vi "Autonics_1Scan.vi"() -> ()   [LabVIEW 2018]
uses:
  <vilib>/Platform/NI_3dgraph.lvlib
  <vilib>/Utility/file.llb/Write To Spreadsheet File (DBL).vi
  <vilib>/DAQmx/read.llb/DAQmx Read (Analog 2D DBL NChan NSamp).vi
  <resource>/objmgr/daqmx.rc
  <vilib>/Instr/_visa.llb/VISA Configure Serial Port (Instr).vi
  <vilib>/Utility/file.llb/Read From Spreadsheet File (DBL).vi
  <vilib>/DAQmx/configure/timing.llb/DAQmx Timing (Sample Clock).vi
  <vilib>/DAQmx/create/channels.llb/DAQmx Create Channel (AI-Voltage-Basic).vi
  <vilib>/Analysis/Matrix/Datatypes/RealMatrix.ctl
  <vilib>/Analysis/Matrix/NI_Matrix.lvlib
panel:
  out "Numeric 2":i32
  out "Numeric":i32
  out "Process Output (Matrix)":T1
  out "Waveform Graph":dbl[](graph)
  in  "Selected Scanning Channel":dbl
  in  "Display Scanning Channel":bool
  out "Waveform Chart":dbl[][](graph)
  in  "Test Channel":bool
  in  "Open":bool
  in  "Scan Distance":dbl=457.0
  in  "Multiplier":dbl=10.0
  in  "Save Button":bool
  in  "No Save":bool
  in  "Save Link":path
  in  "ViewMode":i32(ring) items=["cwViewXYPlane", "cwViewXZPlane", "cwViewYZPlane", "cwViewUserDefined"]
  in  "Back data":bool
  in  "Data Type":u16(ring)=1 items=["Normal", "dX", "dY"]
  in  "Sampling Rate(Hz)":dbl=15000.0
  in  "Samples per Channels":i32=1000
  in  "Min Volts":dbl=-10.0 format="%0.2f"
  in  "Max Volts":dbl=10.0 format="%0.2f"
  in  "Channels":tag="Dev2/ai0:67"
  in  "Scan Step (mm)":dbl=1.0
  in  "Scan":bool
  in  "Plot style":i32(ring)=5 items=["cwLine"=1, "cwPoint"=2, "cwLinePoint"=3, "cwHiddenLine"=4, "cwSurface"=5, "cwSurfaceLine"=6, "cwSurfaceNormal"=7, "cwContourLine"=8, "cwSurfaceContour"=9]
  in  "3D Surface":refnum<k7>(container)
  in  "Flow control":u16(ring) items=["None", "XON/XOFF", "RTS/CTS", "XON/XOFF & RTS/CTS", "DTR/DSR", "XON/XOFF & DTR/DSR"]
  in  "Stop bits":u16(ring)=10 items=["1.0"=10, "1.5"=15, "2.0"=20]
  in  "Parity":dbl
  in  "Data bits":u16=8 min=5 max=8 step=1
  in  "Baud Rate":u32=57600
  in  "COM Port":refnum<visa-resource-name>="COM3"
  in  "Travel per Pulse (mm)":dbl=0.002
  in  "Speed (mm/s)":dbl=5.0
  out "Current  Position (mm)":dbl format="%#_4g"
  in  "Move Distance (mm)":dbl=1.0
  in  "Stop Scan":bool
  in  "Stop":bool
  in  "Home":bool
  in  "Right":bool
  in  "Left":bool
  # "SCANER CONTROL"
  # "BOBBIN MAGNETIC CAMERA"
  # "CHANNELS"
  # "COM Setting"
  # "TIMING"
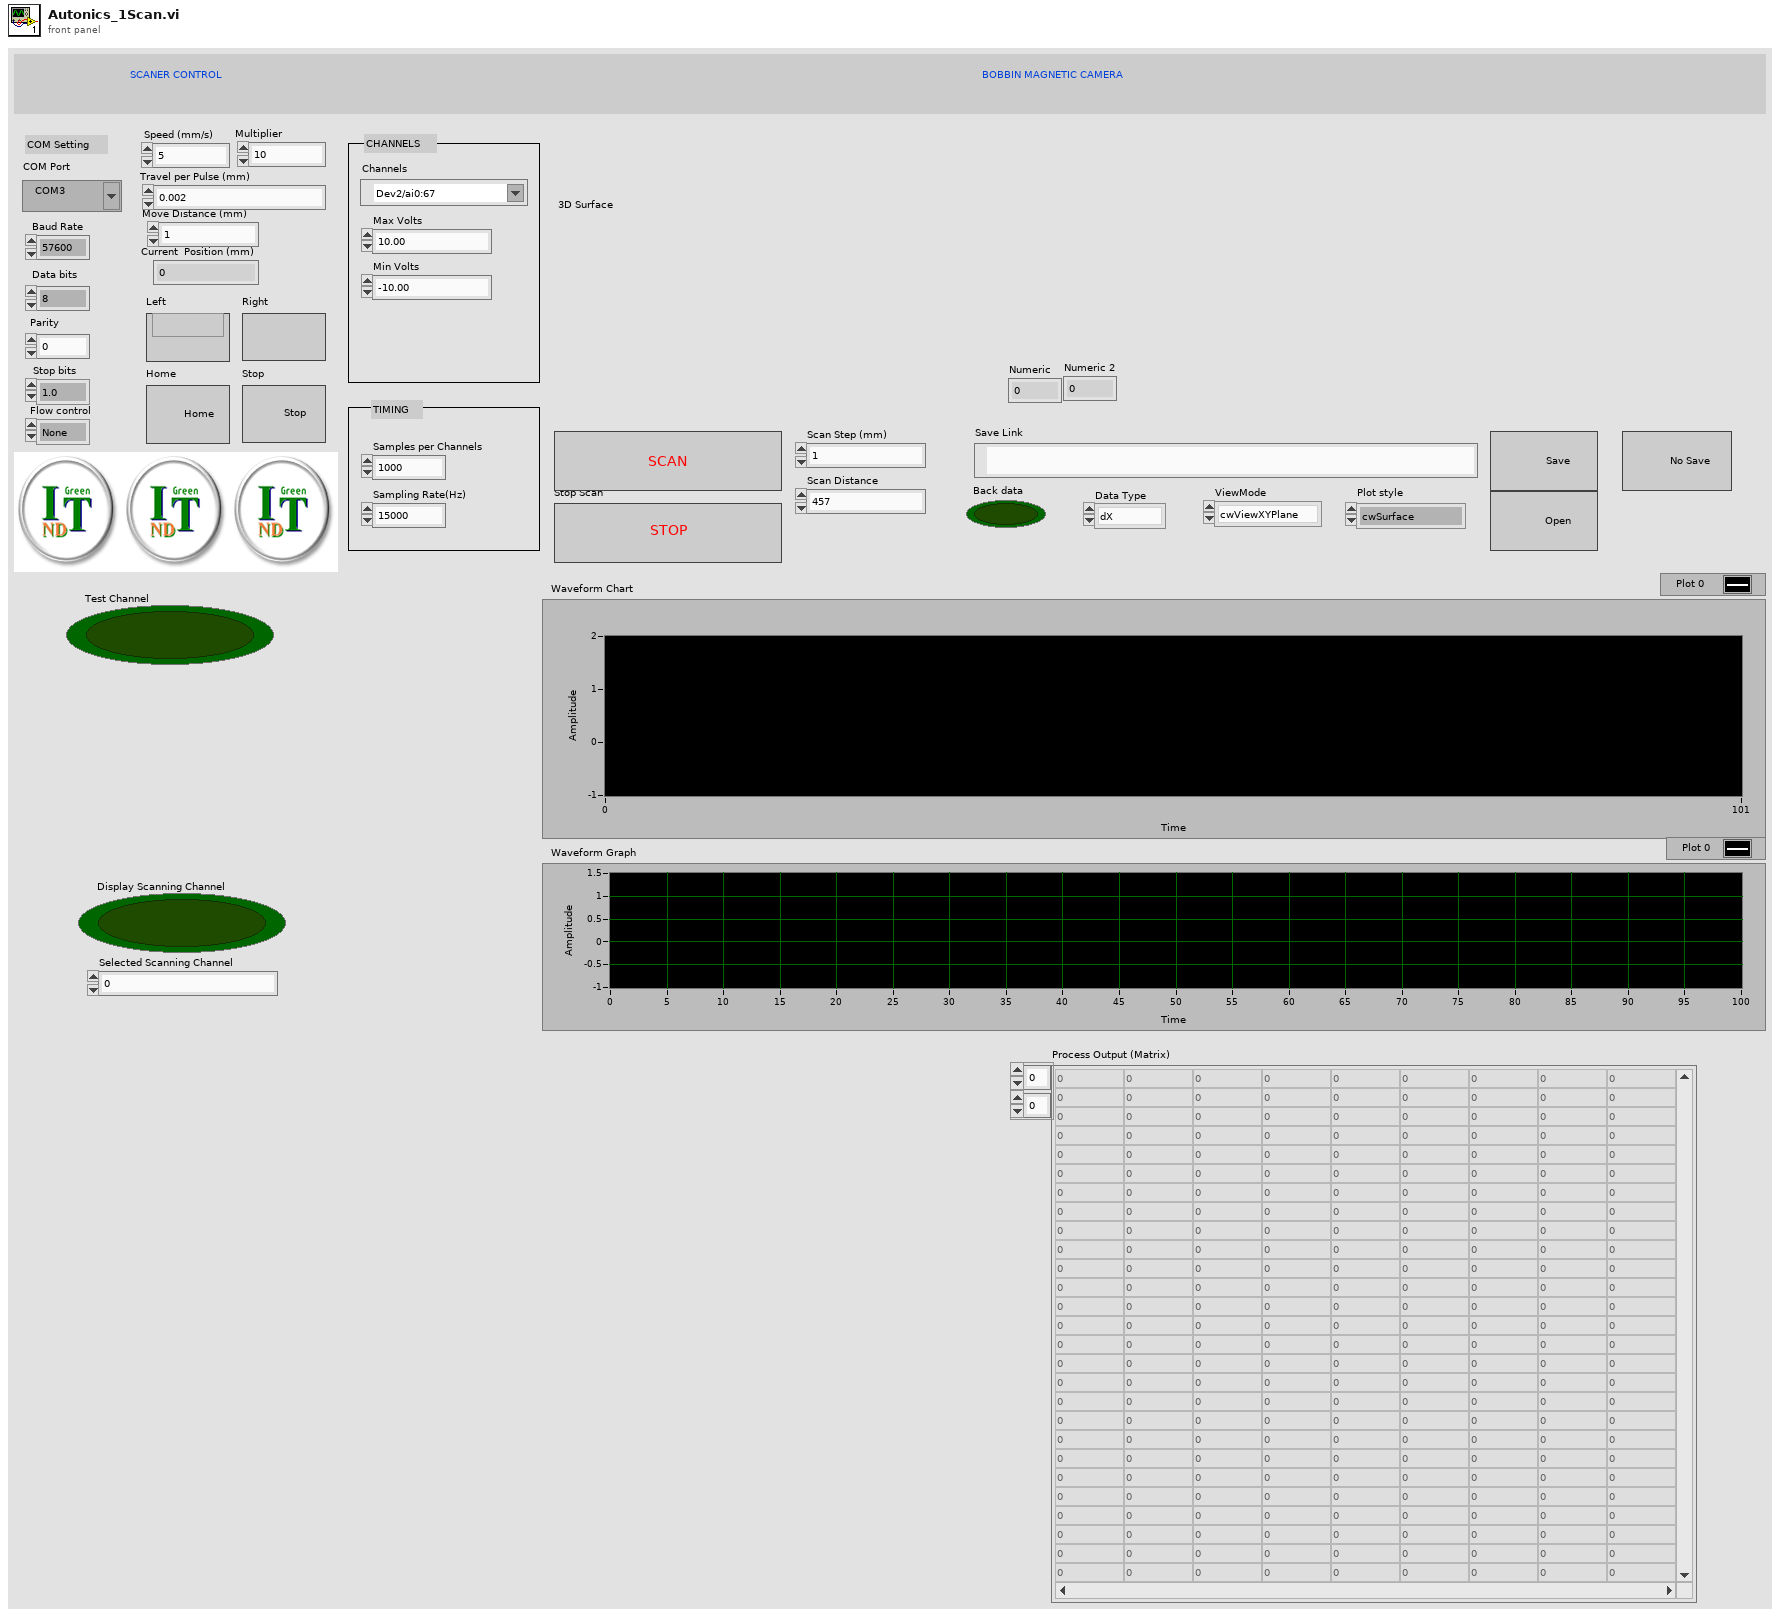
[diagram p1: front panel]
types:
  T1 = typedef "NI_Matrix.lvlib/RealMatrix.ctl" = dbl[][]
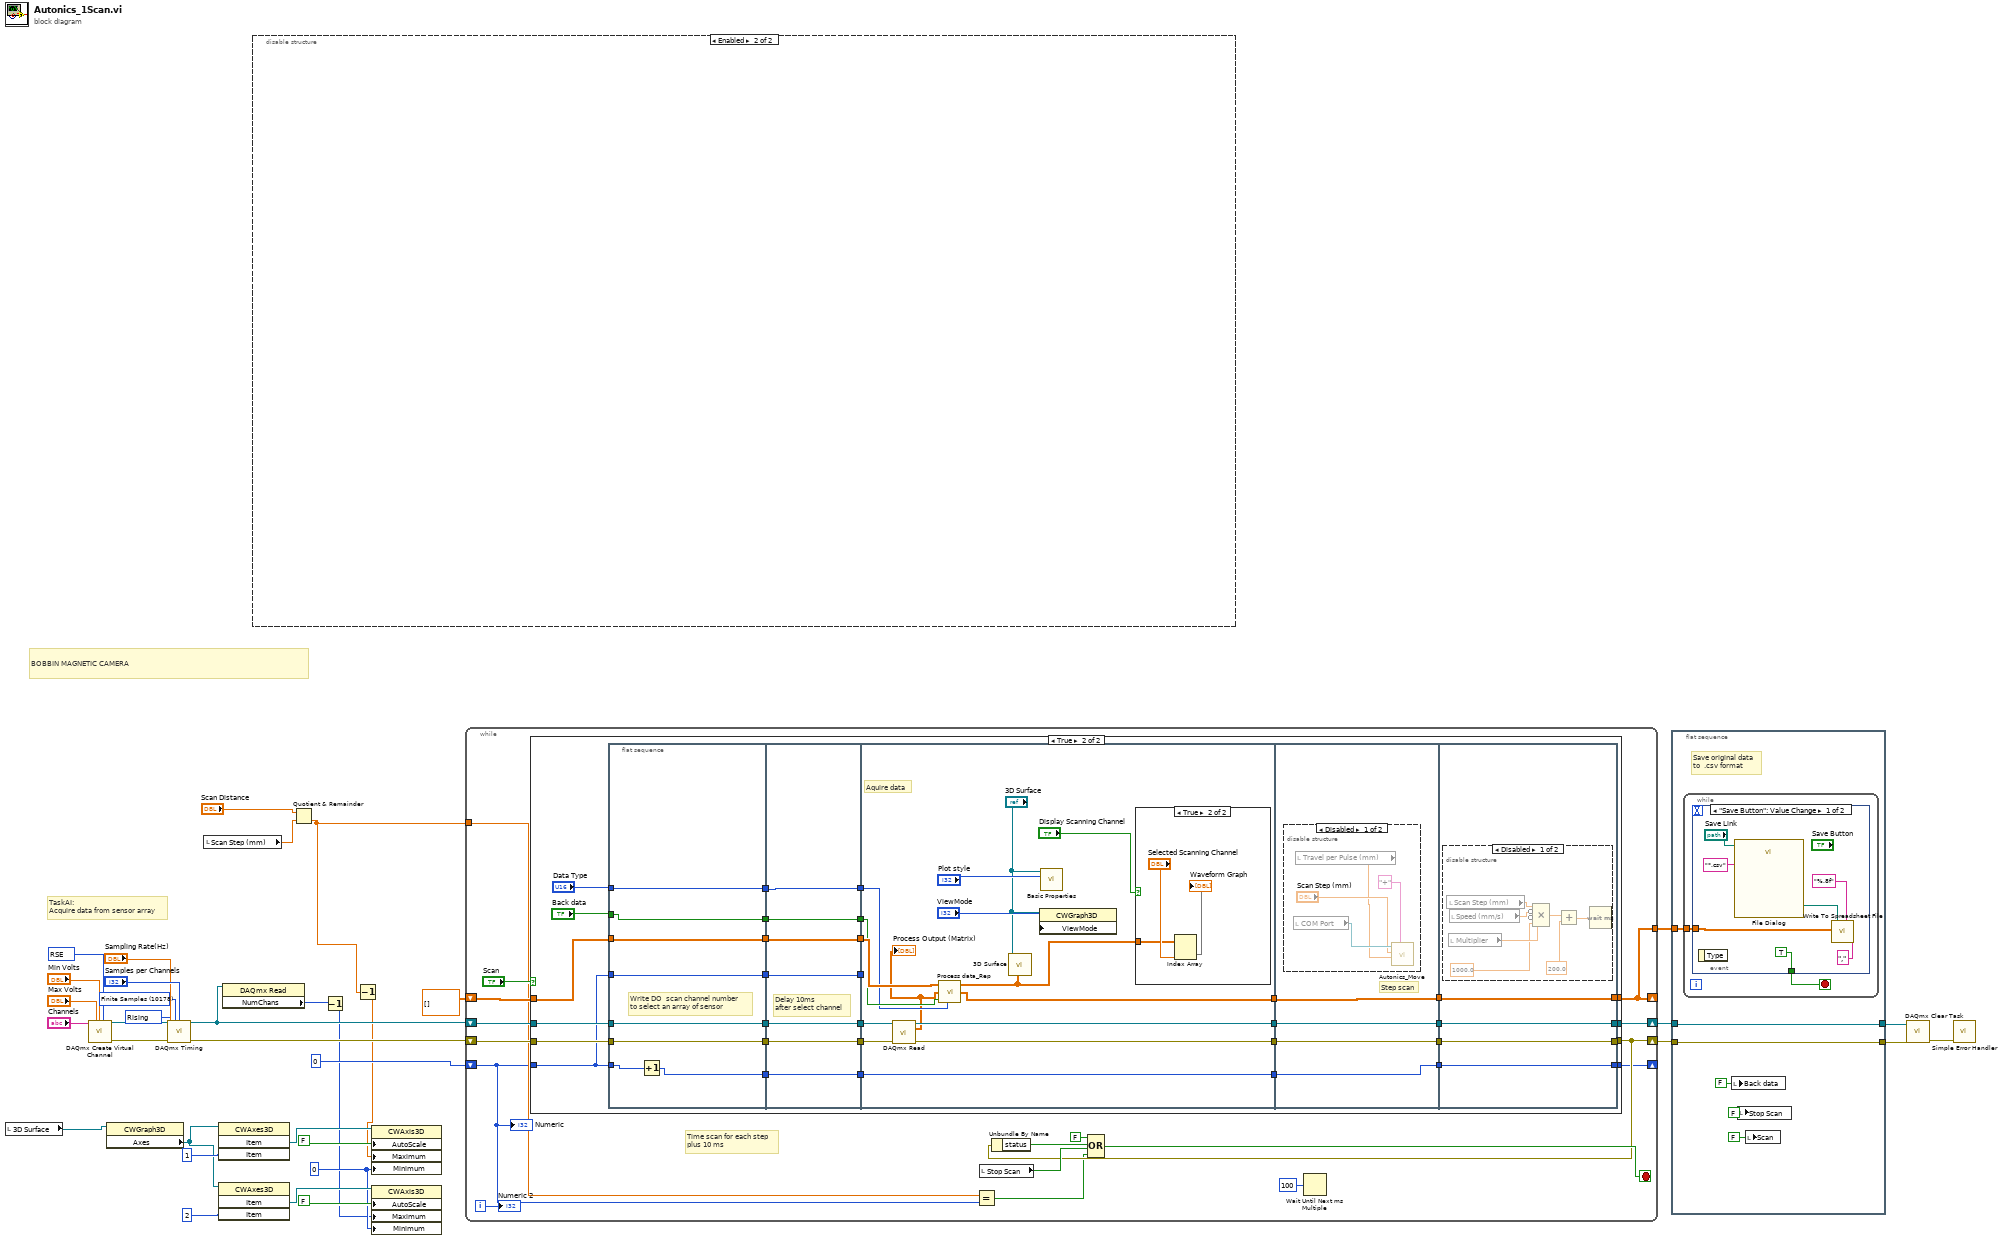
[diagram p0: block diagram]
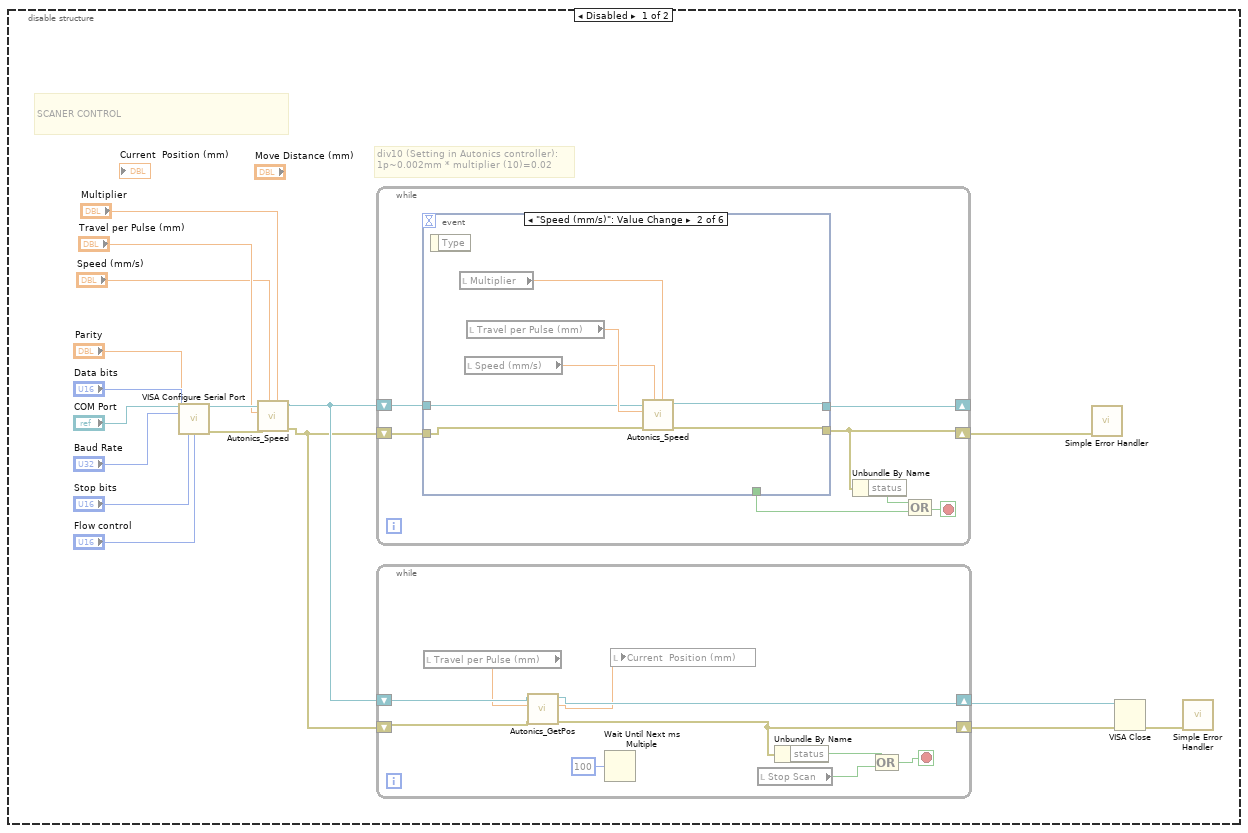
[diagram p2: hidden frame]
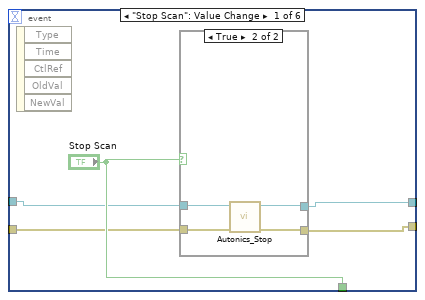
[diagram p3: hidden frame]
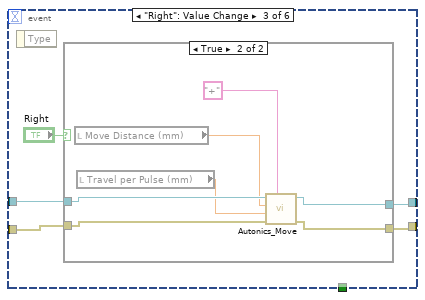
[diagram p5: hidden frame]
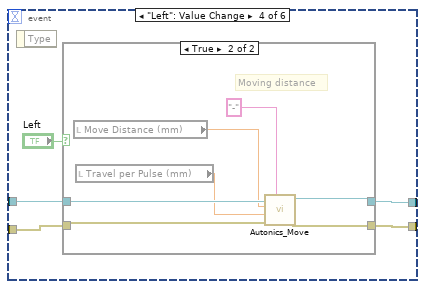
[diagram p7: hidden frame]
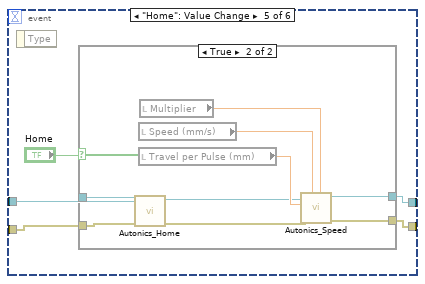
[diagram p9: hidden frame]
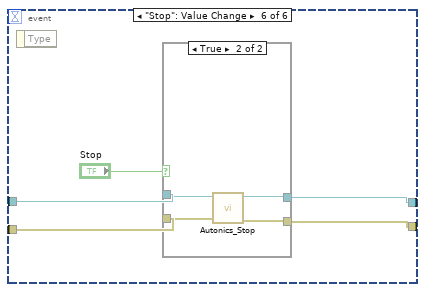
[diagram p11: hidden frame]
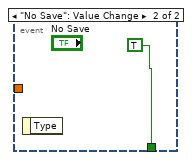
[diagram p13: hidden frame]
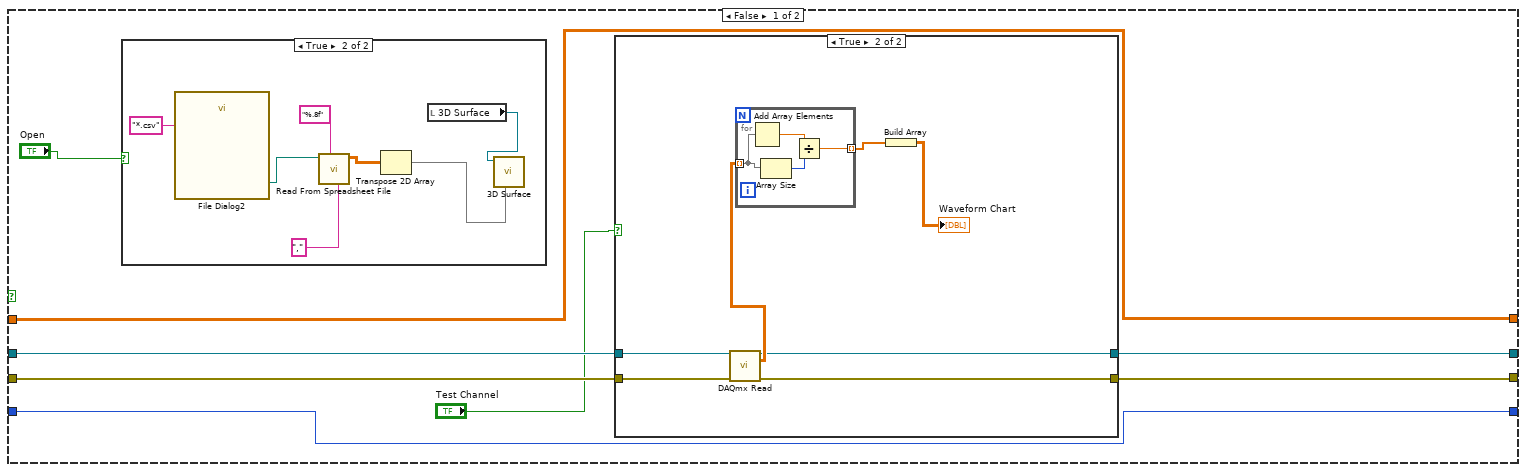
[diagram p14: hidden frame]
diagram:
  w2 = 10280 items=["Rising"=10280, "Falling"=10171] ("active edge")
  w13 = 0
  w26 = 10083 items=["default"=-1, "RSE"=10083, "NRSE"=10078, "Differential"=10106, "Pseudodifferential"=12529] ("input terminal configuration")
  w27 = 10178 items=["Finite Samples"=10178, "Continuous Samples"=10123, "Hardware Timed Single Point"=12522] ("sample mode")
  # "TaskAI:\nAcquire data from sensor array"
  # "BOBBIN MAGNETIC CAMERA"
  n1 = local read "3D Surface"() -> (w21:refnum<k7>)
  n2 = call-poly <vilib>:"DAQmx Create Virtual Channel.vi"("maximum value"="Max Volts", "minimum value"="Min Volts", "input terminal configuration"=w26, "physical channels"="Channels") -> ("task out"=w35:refnum<k21>, "error out"=w34:errorcluster)  [unwired: 10 in]
  n3 = property class="CWGraph3D"(reference=w21) -> ("Axes"=w14:refnum<k7>)  [unwired: 1 in, 2 out]
  n4 = call-poly <vilib>:"DAQmx Timing.vi"("task/channels in"=w35, "sample mode"=w27, "samples per channel"="Samples per Channels", "rate"="Sampling Rate(Hz)", "active edge"=w2, "error in"=w34) -> ("task out"=w25:refnum<k21>, "error out"=w28:errorcluster)  [unwired: 8 in]
  n5 = local read "Scan Step (mm)"() -> (w24:dbl)
  n6 = invoke class="CWAxes3D" method="Item"(reference=w14, "Item"=1) -> ("Item"=w20:refnum<k7>)  [unwired: 2 in, 3 out]
  n7 = invoke class="CWAxes3D" method="Item"(reference=w14, "Item"=2) -> ("Item"=w15:refnum<k7>)  [unwired: 2 in, 3 out]
  n8 = property class="DAQmx Read"(reference=w25) -> ("NumChans"=w4:u32)  [unwired: 1 in, 2 out]
  n9 = disable-structure shown="Enabled" {
    frame Disabled {
      # "div10 (Setting in Autonics controller):\n1p~0.002mm * multiplier (10)=0.02"
      # "SCANER CONTROL"
      n10 = call-poly "VISA Configure Serial Port"("VISA resource name"="COM Port", "baud rate (9600)"="Baud Rate", "data bits (8)"="Data bits", "parity (0:none)"="Parity", "stop bits (10: 1 bit)"="Stop bits", "flow control (0:none)"="Flow control") -> ("VISA resource name out"=w40:refnum<visa-resource-name>, "error out"=w39:errorcluster)  [unwired: 8 in]
      n11 = call "Autonics_Speed.vi"("Multiplier"="Multiplier", "Speed (mm/s)"="Speed (mm/s)", "error in (no error)"=w39, "Travel per  Pulse"="Travel per Pulse (mm)", "VISA resource name"=w40) -> ("error out"=w41:errorcluster, "VISA resource name out"=w42:refnum<visa-resource-name>)  [unwired: 5 in]
      n12 = while {
        shift-right: [w69] -> _
        shift-left: w42 -> [w68]
        shift-right: [w65] -> w45
        shift-left: w41 -> [w67]
        stop <- w64 stop-if-true
        n13 = event shown="[1] \"Speed (mm/s)\": Value Change" {
          selector: _ -> [_ _ _ _ _ _]
          dyn-events: _ -> [_ _ _ _ _ _]
          timeout: _ -> [_ _ _ _ _ _]
          tunnel: w68 -> [w73 w86 w90 w104 w120 w134]
          tunnel: w67 -> [w72 w85 w89 w103 w119 w133]
          tunnel: [w71 w84 w92 w106 w117 w136] -> w69
          tunnel: [w70 w83 w91 w105 w116 w135] -> w65
          tunnel: ["Stop Scan" _ _ _ _ _] -> w63
          event "Stop Scan": Value Change {
            n14 = event-data() -> ()  [unwired: 1 in, 5 out]
            n15 = case shown="True" "Stop Scan" {
              tunnel: [w76 w79] -> w71
              tunnel: [w75 w80] -> w70
              tunnel: w73 -> [w76 w78]
              tunnel: w72 -> [w75 w77]
              frame False {
              }
              frame True {
                n16 = call "Autonics_Stop.vi"("error in (no error)"=w77, "VISA resource name"=w78) -> ("error out"=w80:errorcluster, "VISA resource name out"=w79:refnum<visa-resource-name>)  [unwired: 8 in]
              }
            }
          }
          event "Speed (mm/s)": Value Change {
            n17 = event-data() -> ()  [unwired: 1 in, 1 out]
            n18 = local read "Multiplier"() -> (w81:dbl)
            n19 = local read "Speed (mm/s)"() -> (w82:dbl)
            n20 = local read "Travel per Pulse (mm)"() -> (w87:dbl)
            n21 = call "Autonics_Speed.vi"("Multiplier"=w81, "Speed (mm/s)"=w82, "error in (no error)"=w85, "Travel per  Pulse"=w87, "VISA resource name"=w86) -> ("error out"=w83:errorcluster, "VISA resource name out"=w84:refnum<visa-resource-name>)  [unwired: 5 in]
          }
          event "Right": Value Change {
            n22 = event-data() -> ()  [unwired: 1 in, 1 out]
            n23 = case shown="True" "Right" {
              tunnel: [w93 w99] -> w92
              tunnel: [w94 w98] -> w91
              tunnel: w90 -> [w93 w101]
              tunnel: w89 -> [w94 w100]
              frame False {
              }
              frame True {
                n24 = local read "Move Distance (mm)"() -> (w97:dbl)
                n25 = local read "Travel per Pulse (mm)"() -> (w96:dbl)
                n26 = call "Autonics_Move.vi"("Direction (+)"="+", "error in (no error)"=w100, "Travel per Pulse (mm)"=w96, "Move Distance (mm)"=w97, "VISA resource name"=w101) -> ("error out"=w98:errorcluster, "VISA resource name out"=w99:refnum<visa-resource-name>)  [unwired: 5 in]
              }
            }
          }
          event "Left": Value Change {
            n27 = event-data() -> ()  [unwired: 1 in, 1 out]
            n28 = case shown="True" "Left" {
              tunnel: [w108 w113] -> w106
              tunnel: [w107 w112] -> w105
              tunnel: w104 -> [w108 w115]
              tunnel: w103 -> [w107 w114]
              frame False {
              }
              frame True {
                # "Moving distance"
                n29 = local read "Move Distance (mm)"() -> (w110:dbl)
                n30 = local read "Travel per Pulse (mm)"() -> (w109:dbl)
                n31 = call "Autonics_Move.vi"("Direction (+)"="-", "error in (no error)"=w114, "Travel per Pulse (mm)"=w109, "Move Distance (mm)"=w110, "VISA resource name"=w115) -> ("error out"=w112:errorcluster, "VISA resource name out"=w113:refnum<visa-resource-name>)  [unwired: 5 in]
              }
            }
          }
          event "Home": Value Change {
            n32 = event-data() -> ()  [unwired: 1 in, 1 out]
            n33 = case shown="True" "Home" {
              tunnel: [w122 w124] -> w117
              tunnel: [w121 w123] -> w116
              tunnel: w120 -> [w122 w131]
              tunnel: w119 -> [w121 w130]
              frame False {
              }
              frame True {
                n34 = call "Autonics_Home.vi"("error in (no error)"=w130, "VISA resource name"=w131) -> ("error out"=w125:errorcluster, "VISA resource name out"=w126:refnum<visa-resource-name>)  [unwired: 8 in]
                n35 = local read "Speed (mm/s)"() -> (w128:dbl)
                n36 = local read "Travel per Pulse (mm)"() -> (w129:dbl)
                n37 = local read "Multiplier"() -> (w127:dbl)
                n38 = call "Autonics_Speed.vi"("Multiplier"=w127, "Speed (mm/s)"=w128, "error in (no error)"=w125, "Travel per  Pulse"=w129, "VISA resource name"=w126) -> ("error out"=w123:errorcluster, "VISA resource name out"=w124:refnum<visa-resource-name>)  [unwired: 5 in]
              }
            }
          }
          event "Stop": Value Change {
            n39 = event-data() -> ()  [unwired: 1 in, 1 out]
            n40 = case shown="True" "Stop" {
              tunnel: [w138 w139] -> w136
              tunnel: [w137 w142] -> w135
              tunnel: w134 -> [w138 w141]
              tunnel: w133 -> [w137 w140]
              frame False {
              }
              frame True {
                n41 = call "Autonics_Stop.vi"("error in (no error)"=w140, "VISA resource name"=w141) -> ("error out"=w142:errorcluster, "VISA resource name out"=w139:refnum<visa-resource-name>)  [unwired: 8 in]
              }
            }
          }
        }
        n42 = Unbundle By Name(w65) -> ("status"=w66:bool)
        n43 = Compound Arithmetic op=OR(w66, w63) -> (w64:bool)
      }
      n44 = while {
        shift-right: [w56] -> w44
        shift-left: w42 -> [w58]
        shift-right: [w55] -> w43
        shift-left: w41 -> [w57]
        stop <- w59 stop-if-true
        n45 = local read "Travel per Pulse (mm)"() -> (w54:dbl)
        n46 = call "Autonics_GetPos.vi"("error in (no error)"=w57, "Travel per Pulse (mm)"=w54, "VISA resource name"=w58) -> ("error out"=w55:errorcluster, "Current  Position (mm)"=w53:dbl, "VISA resource name out"=w56:refnum<visa-resource-name>)  [unwired: 6 in]
        n47 = Wait Until Next ms Multiple(millisecond multiple=u32 100) -> ()  [unwired: 1 out]
        n48 = local write "Current  Position (mm)"(w53) -> ()
        n49 = local read "Stop Scan"() -> (w60:bool)
        n50 = Unbundle By Name(w55) -> ("status"=w61:bool)
        n51 = Compound Arithmetic op=OR(w61, w60) -> (w59:bool)
      }
      n52 = call <vilib>:"Simple Error Handler.vi"("error in (no error)"=w45) -> ()  [unwired: 4 in, 5 out]
      n53 = VISA Close(VISA resource name=w44, error in (no error)=w43) -> (error out=w48:errorcluster)
      n54 = call <vilib>:"Simple Error Handler.vi"("error in (no error)"=w48) -> ()  [unwired: 4 in, 5 out]
    }
    frame Enabled {
    }
  }
  n55 = Quotient & Remainder(x="Scan Distance", y=w24) -> (floor(x/y)=w3:dbl)  [unwired: 1 out]
  n56 = Decrement(x=w4) -> (x-1=w12:u32)
  n57 = Decrement(x=w3) -> (x-1=w11:dbl)
  n58 = property class="CWAxis3D"(reference=w20, "AutoScale"=FALSE, "Maximum"=w11, "Minimum"=w13) -> ()  [unwired: 1 in, 2 out]
  n59 = property class="CWAxis3D"(reference=w15, "AutoScale"=FALSE, "Maximum"=w12, "Minimum"=w13) -> ()  [unwired: 1 in, 2 out]
  n60 = while {
    shift-right: [w150] -> _
    shift-left: T1 [] ("Output (Matrix)") -> [w158]
    shift-right: [w156] -> w9
    shift-left: w25 -> [w157]
    shift-right: [w152] -> w7
    shift-left: w28 -> [w159]
    tunnel: [w150] -> w5
    shift-right: [w149] -> _
    shift-left: 0 -> [w147]
    tunnel: w3 -> [w148]
    i -> [w143]
    stop <- w155 stop-if-true
    # "Time scan for each step\nplus 10 ms"
    n61 = case shown="True" "Scan" {
      tunnel: w157 -> [w166 w219]
      tunnel: w159 -> [w164 w218]
      tunnel: w158 -> [w161 w217]
      tunnel: [w165 w213] -> w156
      tunnel: [w163 w212] -> w152
      tunnel: [w161 w211] -> w150
      tunnel: [w162 w198] -> w149
      tunnel: w147 -> [w162 w194]
      frame False {
        n62 = case shown="True" "Open" {
          frame False {
          }
          frame True {
            n63 = call "File Dialog2"("pattern (all files)"="*.csv") -> ("selected path"=w184:path)  [unwired: 11 in, 3 out]
            n64 = call-poly <vilib>:"Read From Spreadsheet File.vi"("delimiter (\\t)"="," ("delimiter (\\t)"), "format (%.3f)"="%.8f", "file path (dialog if empty)"=w184) -> ("all rows"=w182:dbl[][])  [unwired: 4 in, 4 out]
            n65 = Transpose 2D Array(2D array=w182) -> (transposed array=w181:dbl[][])
            n66 = local read "3D Surface"() -> (w185:refnum<k7>)
            n67 = call <vilib>:"3D Surface.vi"("z matrix"=w181, "3D graph"=w185) -> ()  [unwired: 8 in, 2 out]
          }
        }
        n68 = case shown="True" "Test Channel" {
          tunnel: w166 -> [w169 w175]
          tunnel: [w169 w174] -> w165
          tunnel: w164 -> [w168 w173]
          tunnel: [w168 w172] -> w163
          frame False {
          }
          frame True {
            n69 = call-poly <vilib>:"DAQmx Read.vi"("task/channels in"=w175, "error in"=w173) -> ("task out"=w174:refnum<k21>, "data"=w176:dbl[][], "error out"=w172:errorcluster)  [unwired: 11 in]
            n70 = for {
              tunnel: [w179] -> w170 mode=indexing
              tunnel: w176 -> [w177] mode=indexing
              n71 = Add Array Elements(numeric array=w177) -> (sum=w180:dbl)
              n72 = Array Size(array=w177) -> (size(s)=w178:i32)
              n73 = Divide(x=w180, y=w178) -> (x/y=w179:dbl)
            }
            n74 = Build Array(w170) -> (→"Waveform Chart":dbl[][])
          }
        }
      }
      frame True {
        n75 = flat-sequence {
          tunnel: w217 -> [w225]
          tunnel: w218 -> [w226]
          tunnel: w219 -> [w227]
          tunnel: [w227] -> w210
          tunnel: [w226] -> w208
          tunnel: [w225] -> w206
          tunnel: "Back data" -> [w224]
          tunnel: [w224] -> w202
          tunnel: [w223] -> w201
          tunnel: "Data Type" -> [w223]
          tunnel: [w221] -> w195
          tunnel: w194 -> [w222]
          tunnel: w194 -> [w220]
          tunnel: [w220] -> w193
          tunnel: w210 -> [w234]
          tunnel: [w234] -> w209
          tunnel: w208 -> [w233]
          tunnel: [w233] -> w207
          tunnel: w206 -> [w232]
          tunnel: [w232] -> w205
          tunnel: [w231] -> w203
          tunnel: w202 -> [w231]
          tunnel: w201 -> [w230]
          tunnel: [w230] -> w199
          tunnel: [w229] -> w196
          tunnel: w195 -> [w229]
          tunnel: w193 -> [w228]
          tunnel: [w228] -> w192
          tunnel: [w247] -> w216
          tunnel: [w237] -> w215
          tunnel: [w246] -> w214
          tunnel: w209 -> [w249]
          tunnel: w207 -> [w248]
          tunnel: w205 -> [w242]
          tunnel: w203 -> [w241]
          tunnel: w199 -> [w240]
          tunnel: [w239] -> w197
          tunnel: w196 -> [w239]
          tunnel: w192 -> [_]
          tunnel: w216 -> [w256]
          tunnel: w215 -> [w255]
          tunnel: w214 -> [w254]
          tunnel: w197 -> [w253]
          tunnel: [w256] -> w191
          tunnel: [w255] -> w190
          tunnel: [w254] -> w189
          tunnel: [w253] -> w188
          tunnel: [w261] -> w198
          tunnel: [w262] -> w212
          tunnel: [w263] -> w211
          tunnel: [w264] -> w213
          tunnel: w191 -> [w264]
          tunnel: w190 -> [w263]
          tunnel: w189 -> [w262]
          tunnel: w188 -> [w261]
          frame #0 {
            # "Write DO  scan channel number\nto select an array of sensor"
            n76 = Increment(x=w222) -> (x+1=w221:i32)
          }
          frame #1 {
            # "Delay 10ms\nafter select channel"
          }
          frame #2 {
            # "Aquire data"
            n77 = call-poly <vilib>:"DAQmx Read.vi"("task/channels in"=w249, "error in"=w248) -> ("task out"=w247:refnum<k21>, "data"=w235:dbl[][], "error out"=w246:errorcluster)  [unwired: 11 in]
            "Process Output (Matrix)" <- w235
            n78 = call "Process data_Rep.vi"("Initial Matrix"=w242, "Input Matrix"=w235, "Back Data"=w241, "Data Type"=w240) -> ("Process Output (Matrix)"=w236:T1, "Output (Matrix)"=w237:T1)  [unwired: 2 in]
            n79 = call <vilib>:"3D Surface.vi"("z matrix"=w236, "3D graph"="3D Surface") -> ()  [unwired: 8 in, 2 out]
            n80 = property class="CWGraph3D"(reference="3D Surface", "ViewMode"="ViewMode") -> ()  [unwired: 1 in, 2 out]
            n81 = call <vilib>:"Basic Properties.vi"("3D graph"="3D Surface", "plot style"="Plot style") -> ()  [unwired: 12 in, 2 out]
            n82 = case shown="True" "Display Scanning Channel" {
              tunnel: w236 -> [_ w251]
              frame False {
              }
              frame True {
                n83 = Index Array(array=w251, index (col)="Selected Scanning Channel") -> (element=→"Waveform Graph":dbl[])  [unwired: 1 in]
              }
            }
          }
          frame #3 {
            # "Step scan"
            n84 = disable-structure shown="Disabled" {
              frame Disabled {
                n85 = local read "COM Port"() -> (w260:refnum<visa-resource-name>)
                n86 = local read "Travel per Pulse (mm)"() -> (w258:dbl)
                n87 = call "Autonics_Move.vi"("Direction (+)"="+", "Travel per Pulse (mm)"=w258, "Move Distance (mm)"="Scan Step (mm)", "VISA resource name"=w260) -> ()  [unwired: 6 in, 2 out]
              }
              frame Enabled {
              }
            }
          }
          frame #4 {
            n88 = disable-structure shown="Disabled" {
              frame Disabled {
                n89 = local read "Scan Step (mm)"() -> (w267:dbl)
                n90 = local read "Multiplier"() -> (w266:dbl)
                n91 = local read "Speed (mm/s)"() -> (w268:dbl)
                n92 = Compound Arithmetic op=MULTIPLY(w267, invert w268, invert w266, 1000.0 ("value")) -> (w269:dbl)
                n93 = Add(x=w269, y=200.0) -> (x+y=w271:dbl)
                n94 = Wait (ms)(milliseconds to wait=w271) -> ()  [unwired: 1 out]
              }
              frame Enabled {
              }
            }
          }
        }
      }
    }
    n95 = Equal?(x=w148, y=w147) -> (x = y?=w146:bool)
    n96 = local read "Stop Scan"() -> (w153:bool)
    n97 = Unbundle By Name(w152) -> ("status"=w151:bool)
    n98 = Compound Arithmetic op=OR(FALSE ("value"), w151, w153, w146) -> (w155:bool)
    n99 = Wait Until Next ms Multiple(millisecond multiple=u32 100) -> ()  [unwired: 1 out]
    "Numeric" <- w147
    "Numeric 2" <- w143
  }
  n100 = flat-sequence {
    tunnel: w9 -> [w277]
    tunnel: [w277] -> w8
    tunnel: w7 -> [w276]
    tunnel: [w276] -> w6
    tunnel: w5 -> [w273]
    frame #0 {
      # "Save original data\nto  .csv format"
      n101 = while {
        tunnel: w273 -> [w279]
        stop <- w278 stop-if-true
        n102 = event shown="[0] \"Save Button\": Value Change" {
          selector: _ -> [_ _]
          dyn-events: _ -> [_ _]
          timeout: _ -> [_ _]
          tunnel: w279 -> [w286 _]
          tunnel: [TRUE TRUE] -> w278
          event "Save Button": Value Change {
            n103 = event-data() -> ()  [unwired: 1 in, 1 out]
            n104 = call "File Dialog"("start path"="Save Link", "pattern (all files)"="*.csv") -> ("selected path"=w282:path)  [unwired: 10 in, 3 out]
            n105 = call-poly <vilib>:"Write To Spreadsheet File.vi"("delimiter (\\t)"="," ("delimiter (\\t)"), "format (%.3f)"="%.8f", "2D data"=w286, "file path (dialog if empty)"=w282) -> ()  [unwired: 4 in, 1 out]
          }
          event "No Save": Value Change {
            n106 = event-data() -> ()  [unwired: 1 in, 1 out]
          }
        }
      }
      n107 = local write "Back data"(FALSE ("Back data")) -> ()
      n108 = local write "Stop Scan"(FALSE ("Exit")) -> ()
      n109 = local write "Scan"(FALSE ("Scan")) -> ()
    }
  }
  n110 = call <vilib>:"DAQmx Clear Task.vi"("task in"=w8, "error in"=w6) -> ("error out"=w10:errorcluster)  [unwired: 13 in]
  n111 = call <vilib>:"Simple Error Handler.vi"("error in (no error)"=w10) -> ()  [unwired: 4 in, 5 out]
